vi "Build Array and Concatenate (2D).vi"(10 "Array":dbl[](array[numeric])) -> (2 "Array Out":dbl[](array[numeric]))   [LabVIEW 2021]
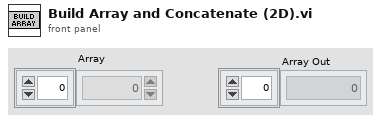
[diagram p1: front panel]
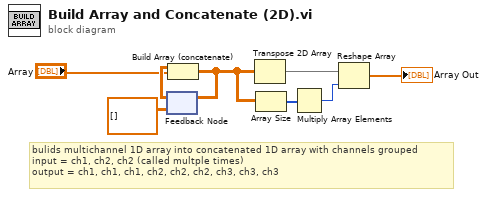
[diagram p0: block diagram]
diagram:
  # "bulids multichannel 1D array into concatenated 1D array with channels grouped\ninput = ch1, ch2, ch2 (called multple times)\noutput = ch1, ch1, ch1, ch2, ch2, ch2, ch3, ch3, ch3"
  n1 = feedback #1(dbl[][] []) -> (w8:dbl[][])
  n2 = Build Array (concatenate)(w8, "Array") -> (w2:dbl[][])
  n3 = feedback-in #1(w2) -> ()
  n4 = Transpose 2D Array(2D array=w2) -> (transposed array=w3:dbl[][])
  n5 = Array Size(array=w2) -> (size(s)=w5:i32[])
  n6 = Multiply Array Elements(1:w5) -> (0:w4:i32)
  n7 = Reshape Array(w3, w4) -> (→"Array Out":dbl[])
